vi "New Name Dialog.vi"(10 "Names":cluster{"String":string, "Value":string}[](array[cluster])) -> (1 "OK":bool, 2 "NamesOut":cluster{"String":string, "Value":string}[](array[cluster]), 3 "NewName":cluster{"String":string, "Value":string})   [LabVIEW 2015]
panel:
  in  "Cancel Button":bool
  in  "OK Button":bool
  in  "NewName":string caption="New Tretment Name"
  # "Please enter a new treatment name."
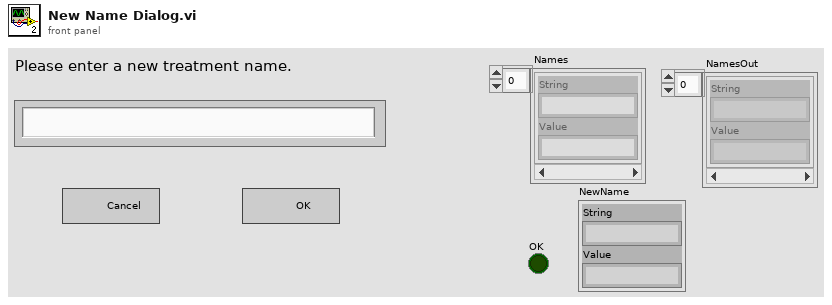
[diagram p1: front panel]
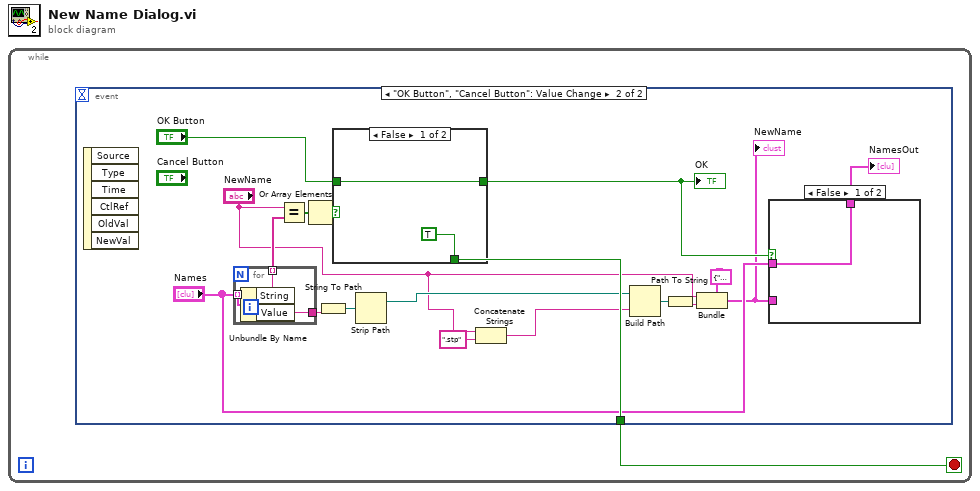
[diagram p0: block diagram]
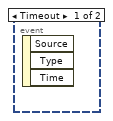
[diagram p2: hidden frame]
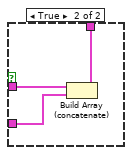
[diagram p3: hidden frame]
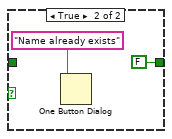
[diagram p4: hidden frame]
diagram:
  n1 = while {
    stop <- w1 stop-if-true
    n2 = event shown="[1] \"OK Button\", \"Cancel Button\": Value Change" {
      selector: _ -> [_ _]
      dyn-events: _ -> [_ _]
      timeout: _ -> [_ _]
      tunnel: [_ w17] -> w1
      event Timeout {
        n3 = event-data() -> ()  [unwired: 1 in, 3 out]
      }
      event "OK Button", "Cancel Button": Value Change {
        n4 = event-data() -> ()  [unwired: 1 in, 6 out]
        n5 = for {
          tunnel: "Names" -> [w26] mode=indexing
          tunnel: [w25] -> w15 mode=indexing
          tunnel: [w24] -> w11
          n6 = Unbundle By Name(w26) -> ("String"=w25:string, "Value"=w24:string)
        }
        n7 = Equal?(x="NewName", y=w15) -> (x = y?=w19:bool[])
        n8 = Or Array Elements(Boolean array=w19) -> (logical OR=w18:bool)
        n9 = String To Path(string=w11) -> (path=w10:path)
        n10 = case shown="False" w18 {
          tunnel: [TRUE _] -> w17
          tunnel: [w27 FALSE ("OK Button")] -> w14
          tunnel: "OK Button" -> [w27 _]
          frame False {
          }
          frame True {
            n11 = One Button Dialog(message="Name already exists") -> ()  [unwired: 1 in, 1 out]
          }
        }
        "OK" <- w14
        n12 = Strip Path(path=w10) -> (stripped path=w9:path)  [unwired: 1 out]
        n13 = Concatenate Strings("NewName", ".stp" ("string")) -> (w2:string)
        n14 = Build Path(base path=w9, name or relative path=w2) -> (appended path=w7:path)
        n15 = Path To String(path=w7) -> (string=w6:string)
        n16 = Bundle(cluster=cluster{"String":string, "Value":string} {"String"="", "Value"=""}, "String"="NewName", "Value"=w6) -> (w5:cluster{"String":string, "Value":string})
        "NewName" <- w5
        n17 = case shown="False" w14 {
          tunnel: "Names" -> [w20 w23]
          tunnel: [w20 w22] -> w12
          tunnel: w5 -> [_ w21]
          frame False {
          }
          frame True {
            n18 = Build Array (concatenate)(w23, w21) -> (w22:cluster{"String":string, "Value":string}[])
          }
        }
        "NamesOut" <- w12
      }
    }
  }
